vi "Read Filter Cycle.vi"(8 "error in (no error)":errorcluster, 11 "Reset cycle state STEP in":refnum<class "Reset cycle state STEP.lvclass">) -> (0 "error out":errorcluster, 2 "Filter Cycle":bool, 3 "Reset cycle state STEP out":refnum<class "Reset cycle state STEP.lvclass">)   [LabVIEW 2014, in "Reset cycle state STEP.lvclass"]
uses:
  Reset cycle state STEP.lvclass
  Reset cycle state STEP.lvclass/Reset cycle state STEP.ctl
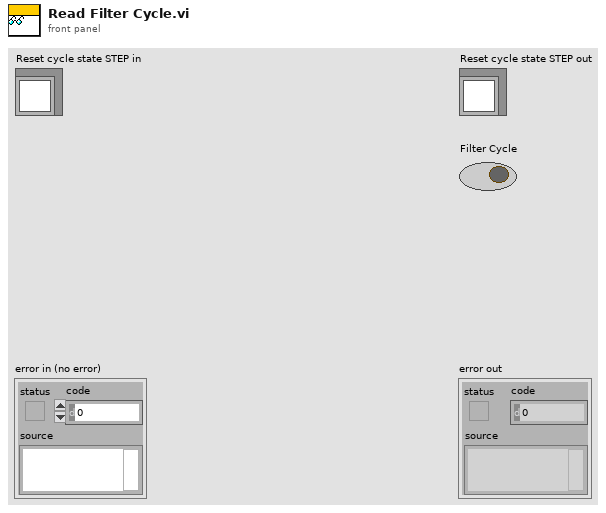
[diagram p1: front panel]
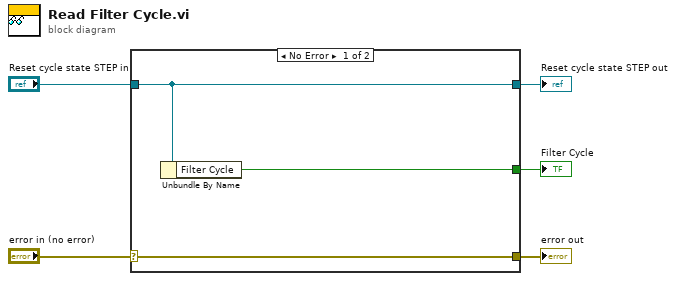
[diagram p0: block diagram]
diagram:
  n1 = case shown="No Error" "error in (no error)" {
    selector: "error in (no error)" -> [w8 w9]
    tunnel: [w8 w9] -> w4
    tunnel: [w7 w10] -> w2
    tunnel: "Reset cycle state STEP in" -> [w7 w10]
    tunnel: [w6 _] -> w1
    frame No Error {
      n2 = Unbundle By Name(w7) -> ("Filter Cycle"=w6:bool)
    }
    frame Error {
    }
  }
  "error out" <- w4
  "Reset cycle state STEP out" <- w2
  "Filter Cycle" <- w1
